vi "Update UI.vi"(8 "error in (no error)":errorcluster, 11 "Model Data in":T1) -> (0 "error out":errorcluster, 3 "Model Data out":T1)   [LabVIEW 2014, in "Model.lvlib"]
uses:
  Model.lvlib
  TypeDefs/PL Settings.ctl
  TypeDefs/PL UI Refs.ctl
  TypeDefs/Model Data.ctl
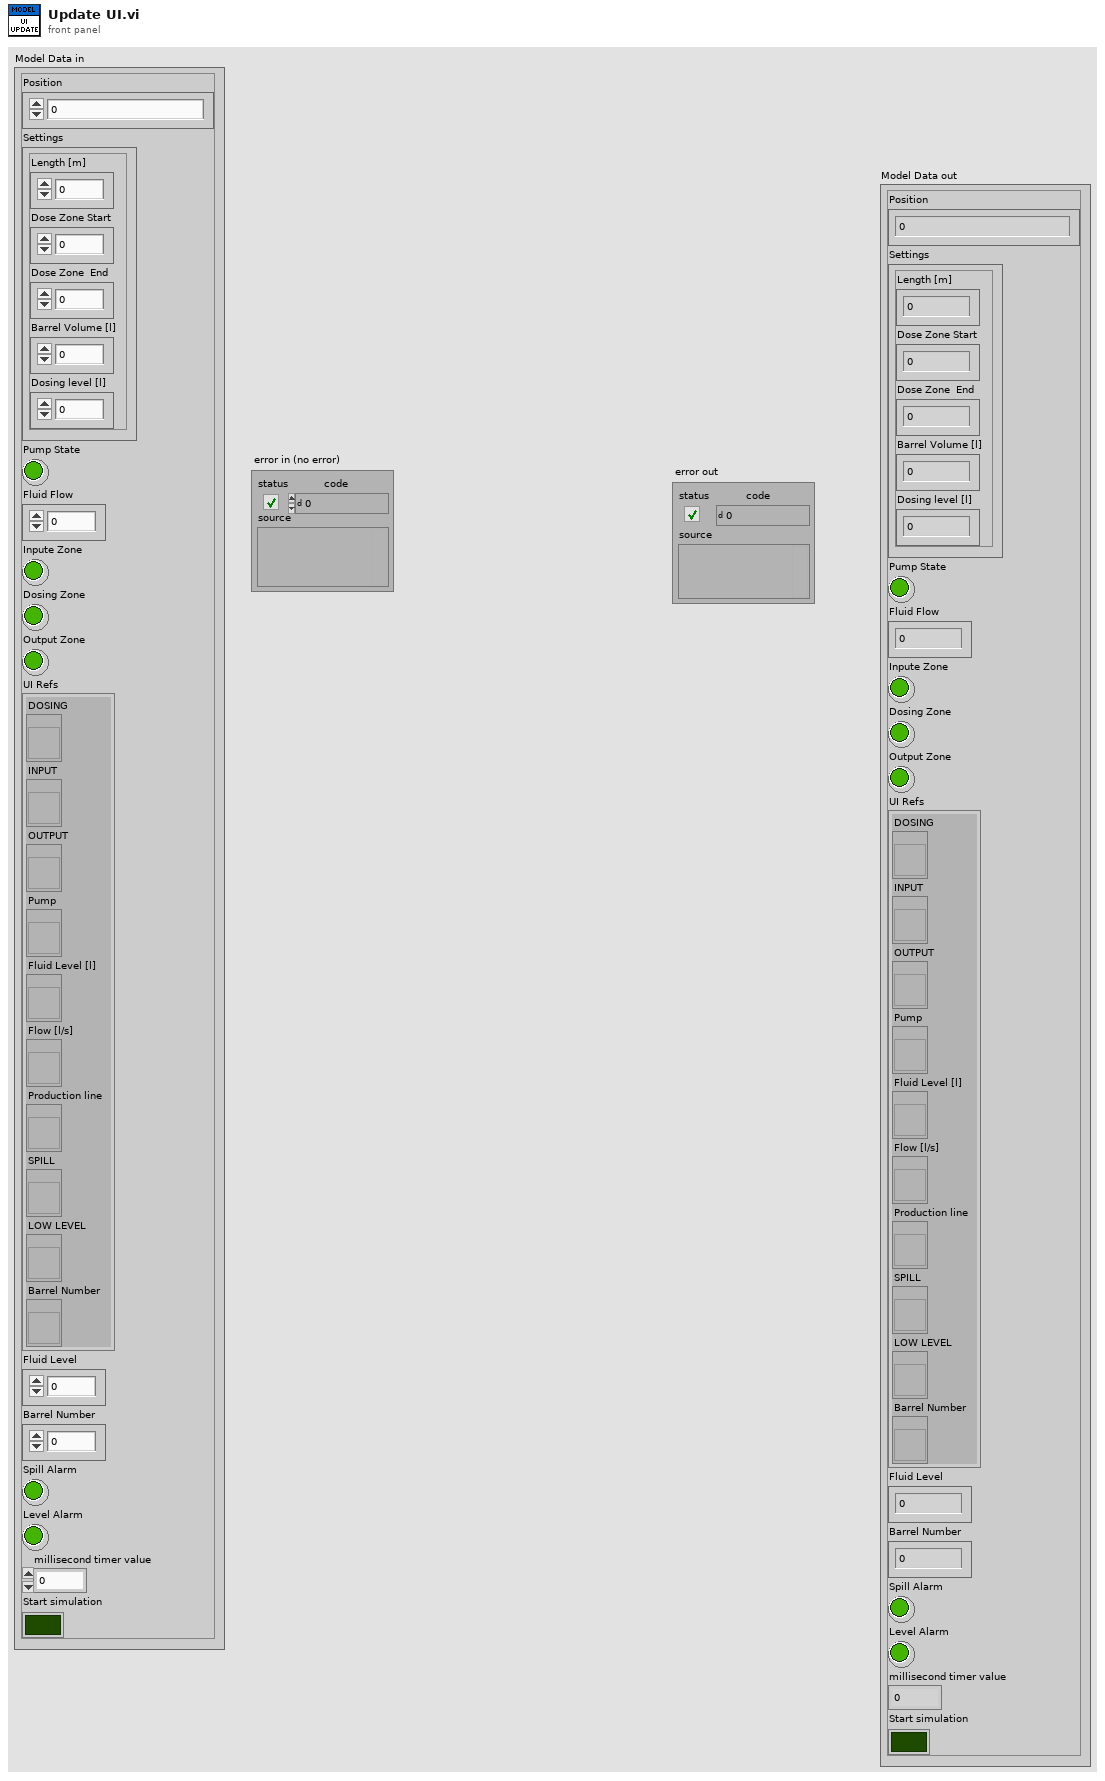
[diagram p1: front panel]
types:
  T1 = typedef "Model.lvlib/Model Data.ctl" = cluster{"Position":dbl, "Settings":T2, "Pump State":bool, "Fluid Flow":dbl, "Inpute Zone":bool, "Dosing Zone":bool, "Output Zone":bool, "UI Refs":T3, "Fluid Level":dbl, "Barrel Number":i32, "Spill Alarm":bool, "Level Alarm":bool, "millisecond timer value":u32, "Start simulation":bool}
  T2 = typedef "Model.lvlib/PL Settings.ctl" = cluster{"Length [m]":dbl, "Dose Zone Start":dbl, "Dose Zone  End":dbl, "Barrel Volume [l]":dbl, "Dosing level [l]":dbl}
  T3 = typedef "Model.lvlib/PL UI Refs.ctl" = cluster{"DOSING":refnum<vi>, "INPUT":refnum<vi>, "OUTPUT":refnum<vi>, "Pump":refnum<vi>, "Fluid Level [l]":refnum<vi>, "Flow [l/s]":refnum<vi>, "Production line":refnum<vi>, "SPILL":refnum<vi>, "LOW LEVEL":refnum<vi>, "Barrel Number":refnum<vi>}
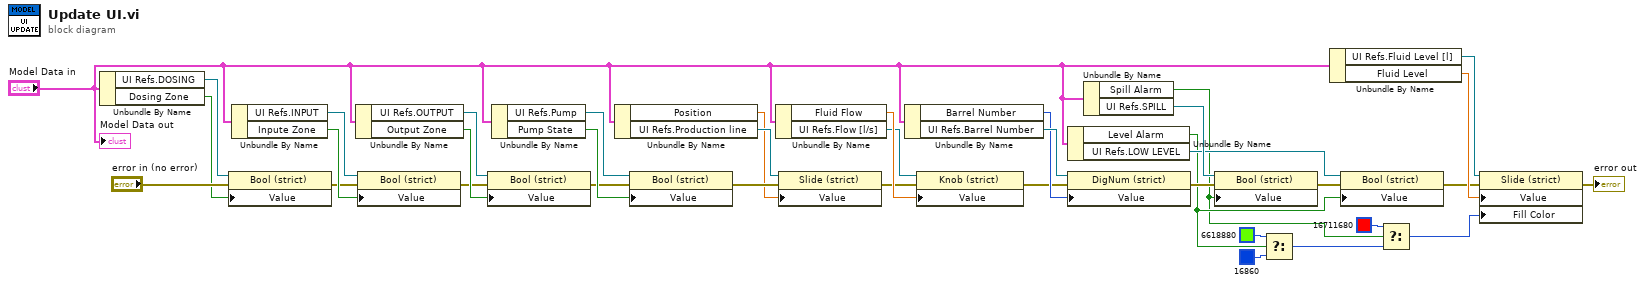
[diagram p0: block diagram]
diagram:
  n1 = Unbundle By Name("Model Data in") -> ("UI Refs.DOSING"=w35:refnum<vi>, "Dosing Zone"=w36:bool)
  n2 = property class="Bool (strict)"(reference=w35, error in="error in (no error)", "Value"=w36) -> (error out=w32:errorcluster)  [unwired: 1 out]
  n3 = Unbundle By Name("Model Data in") -> ("UI Refs.INPUT"=w34:refnum<vi>, "Inpute Zone"=w33:bool)
  n4 = Unbundle By Name("Model Data in") -> ("UI Refs.OUTPUT"=w31:refnum<vi>, "Output Zone"=w30:bool)
  n5 = property class="Bool (strict)"(reference=w34, error in=w32, "Value"=w33) -> (error out=w29:errorcluster)  [unwired: 1 out]
  n6 = property class="Bool (strict)"(reference=w31, error in=w29, "Value"=w30) -> (error out=w26:errorcluster)  [unwired: 1 out]
  n7 = Unbundle By Name("Model Data in") -> ("UI Refs.Pump"=w28:refnum<vi>, "Pump State"=w27:bool)
  n8 = Unbundle By Name("Model Data in") -> ("Position"=w23:dbl, "UI Refs.Production line"=w24:refnum<vi>)
  n9 = property class="Bool (strict)"(reference=w28, error in=w26, "Value"=w27) -> (error out=w25:errorcluster)  [unwired: 1 out]
  n10 = Unbundle By Name("Model Data in") -> ("Fluid Flow"=w14:dbl, "UI Refs.Flow [l/s]"=w13:refnum<vi>)
  n11 = property class="Slide (strict)"(reference=w24, error in=w25, "Value"=w23) -> (error out=w9:errorcluster)  [unwired: 1 out]
  n12 = Unbundle By Name("Model Data in") -> ("Barrel Number"=w19:i32, "UI Refs.Barrel Number"=w20:refnum<vi>)
  n13 = property class="Knob (strict)"(reference=w13, error in=w9, "Value"=w14) -> (error out=w12:errorcluster)  [unwired: 1 out]
  n14 = Unbundle By Name("Model Data in") -> ("Level Alarm"=w7:bool, "UI Refs.LOW LEVEL"=w15:refnum<vi>)
  n15 = property class="DigNum (strict)"(reference=w20, error in=w12, "Value"=w19) -> (error out=w17:errorcluster)  [unwired: 1 out]
  n16 = Unbundle By Name("Model Data in") -> ("Spill Alarm"=w4:bool, "UI Refs.SPILL"=w18:refnum<vi>)
  n17 = property class="Bool (strict)"(reference=w18, error in=w17, "Value"=w4) -> (error out=w16:errorcluster)  [unwired: 1 out]
  n18 = Select(t=u32 6618880, s=w7, f=u32 16860) -> (s? t:f=w3:u32)
  n19 = Unbundle By Name("Model Data in") -> ("UI Refs.Fluid Level [l]"=w22:refnum<vi>, "Fluid Level"=w21:dbl)
  n20 = property class="Bool (strict)"(reference=w15, error in=w16, "Value"=w7) -> (error out=w11:errorcluster)  [unwired: 1 out]
  n21 = Select(t=u32 16711680, s=w4, f=w3) -> (s? t:f=w1:u32)
  n22 = property class="Slide (strict)"(reference=w22, error in=w11, "Value"=w21, "Fill Color"=w1) -> (error out=→"error out":errorcluster)  [unwired: 1 out]
  "Model Data out" <- "Model Data in"
